vi "LCD string VI.vi"(0 "Error In":errorcluster, 1 "Tank Level (L)":dbl, 3 "1 - cm\n2 - L":dbl=1.0 min=1.0 max=2.0) -> ()   [LabVIEW 2017]
uses:
  <vilib>/MakerHub/LINX/Public/Utilities/Open Serial.vi
  <vilib>/MakerHub/LINX/LMH-LINX.lvlib
panel:
  out "Centimeters":dbl
  in  "stop":bool
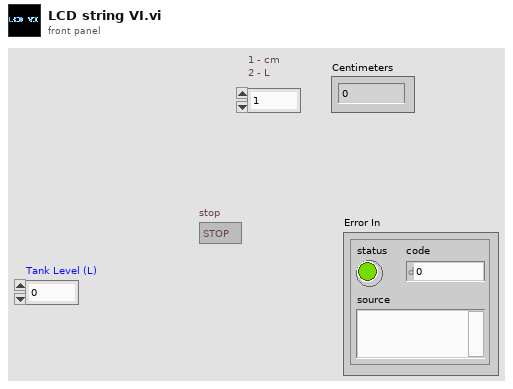
[diagram p1: front panel]
types:
  T1 = typedef "LMH-LINX.lvlib/LINX Ref.ctl" = cluster{"IO":T2, "Interface":T3, "LINX Device Config":T4}
  T2 = typedef "LMH-LINX.lvlib/Platform.ctl" = enum16{"Remote", "Local"}
  T3 = typedef "LMH-LINX.lvlib/Interface.ctl" = enum16{"Serial", "TCP"}
  T4 = typedef "LMH-LINX.lvlib/Device.lvlib/LINX Device Config.ctl" = cluster{"Interface":T3, "COM Port":refnum<visa-resource-name>, "TCP Configuration":T5, "Device Family":u8, "Device ID":u8, "Device Name":string, "TCP Ref":refnum<k5>, "Channels":T6}
  T5 = typedef "LMH-LINX.lvlib/Device.lvlib/TCP Config.ctl" = cluster{"IP Address":string, "Port":u16}
  T6 = typedef "LMH-LINX.lvlib/Channels.ctl" = cluster{"DI":u8[], "DO":u8[], "AI":u8[], "AO":u8[], "PWM":u8[], "QE":u8[], "UART":u8[], "I2C 2":u8[], "SPI":u8[], "CAN":u8[], "Servo":u8[], "AI Ref (V)":dbl, "AI Resolution (Bits)":u8, "AO Ref (V)":dbl, "AO Resolution (Bits)":u8}
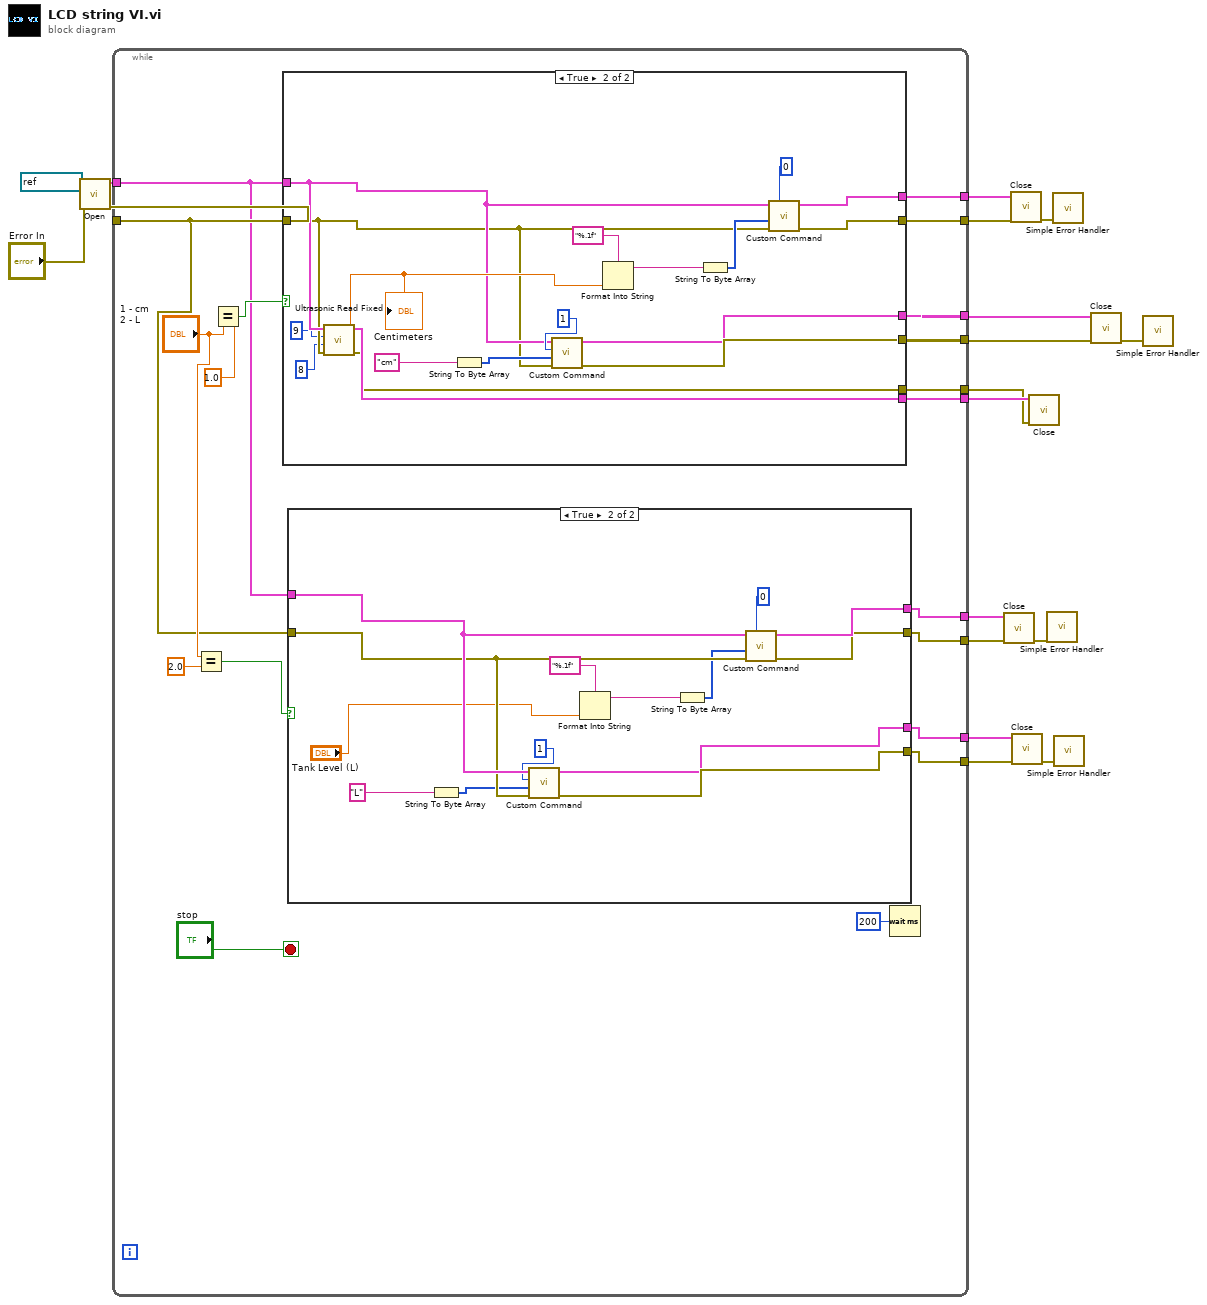
[diagram p0: block diagram]
diagram:
  n1 = call-poly <vilib>:"Open.vi"("Error In"="Error In", "Serial Port"=refnum<visa-resource-name> "COM7") -> ("Error Out"=w15:errorcluster, "LINX Resource"=w14:T1)  [unwired: 7 in, 1 out]
  n2 = while {
    tunnel: w14 -> [w26]
    tunnel: w15 -> [w25]
    tunnel: [w37] -> w18
    tunnel: [w36] -> w17
    tunnel: [w35] -> w12
    tunnel: [w34] -> w11
    tunnel: [w24] -> w8
    tunnel: [w23] -> w7
    tunnel: [w22] -> w6
    tunnel: [w21] -> w5
    tunnel: [w20] -> w2
    tunnel: [w19] -> w1
    stop <- "stop" stop-if-true
    n3 = Equal?(x="1 - cm\n2 - L", y=2.0) -> (x = y?=w27:bool)
    n4 = Equal?(x="1 - cm\n2 - L", y=1.0) -> (x = y?=w30:bool)
    n5 = case shown="True" w30 {
      tunnel: w26 -> [w55 w61]
      tunnel: w25 -> [w54 w60]
      tunnel: [w55 w73] -> w37
      tunnel: [w54 w72] -> w36
      tunnel: [w54 w71] -> w35
      tunnel: [w55 w70] -> w34
      tunnel: [w55 w59] -> w20
      tunnel: [w54 w58] -> w19
      frame False {
      }
      frame True {
        n6 = call "Ultrasonic Read Fixed.vi"("Error In"=w60, "DO Channel"=u8 8, "DI Channel"=u8 9, "LINX Resource"=w61) -> ("Error Out"=w58:errorcluster, "Centimeters"=w62:dbl, "LINX Resource"=w59:T1)  [unwired: 4 in, 1 out]
        "Centimeters" <- w62
        n7 = String To Byte Array(string="cm") -> (unsigned byte array=w66:u8[])
        n8 = call <vilib>:"Custom Command.vi"("Error In"=w60, "Data"=w66, "Custom Command Number"=u16 1, "LINX Resource"=w61) -> ("Error Out"=w71:errorcluster, "LINX Resource"=w70:T1)  [unwired: 4 in, 2 out]
        n9 = Format Into String(format string="%.1f", w62) -> (resulting string=w68:string)  [unwired: 2 in, 1 out]
        n10 = String To Byte Array(string=w68) -> (unsigned byte array=w67:u8[])
        n11 = call <vilib>:"Custom Command.vi"("Error In"=w60, "Data"=w67, "Custom Command Number"=u16 0, "LINX Resource"=w61) -> ("Error Out"=w72:errorcluster, "LINX Resource"=w73:T1)  [unwired: 4 in, 2 out]
      }
    }
    n12 = case shown="True" w27 {
      tunnel: w26 -> [w39 w53]
      tunnel: w25 -> [w38 w52]
      tunnel: [w39 w51] -> w24
      tunnel: [w38 w50] -> w23
      tunnel: [w38 w49] -> w21
      tunnel: [w39 w48] -> w22
      frame False {
      }
      frame True {
        n13 = String To Byte Array(string="L") -> (unsigned byte array=w44:u8[])
        n14 = call <vilib>:"Custom Command.vi"("Error In"=w52, "Data"=w44, "Custom Command Number"=u16 1, "LINX Resource"=w53) -> ("Error Out"=w49:errorcluster, "LINX Resource"=w48:T1)  [unwired: 4 in, 2 out]
        n15 = Format Into String(format string="%.1f", "Tank Level (L)") -> (resulting string=w46:string)  [unwired: 2 in, 1 out]
        n16 = String To Byte Array(string=w46) -> (unsigned byte array=w45:u8[])
        n17 = call <vilib>:"Custom Command.vi"("Error In"=w52, "Data"=w45, "Custom Command Number"=u16 0, "LINX Resource"=w53) -> ("Error Out"=w50:errorcluster, "LINX Resource"=w51:T1)  [unwired: 4 in, 2 out]
      }
    }
    n18 = Wait (ms)(milliseconds to wait=u32 200) -> ()  [unwired: 1 out]
  }
  n19 = call <vilib>:"Close.vi"("Error In"=w7, "LINX Resource"=w8) -> ("Error Out"=w10:errorcluster)  [unwired: 9 in]
  n20 = call <vilib>:"Close.vi"("Error In"=w17, "LINX Resource"=w18) -> ("Error Out"=w16:errorcluster)  [unwired: 9 in]
  n21 = call <vilib>:"Close.vi"("Error In"=w5, "LINX Resource"=w6) -> ("Error Out"=w9:errorcluster)  [unwired: 9 in]
  n22 = call <vilib>:"Close.vi"("Error In"=w1, "LINX Resource"=w2) -> ()  [unwired: 9 in, 1 out]
  n23 = call <vilib>:"Simple Error Handler.vi"("error in (no error)"=w10) -> ()  [unwired: 4 in, 5 out]
  n24 = call <vilib>:"Simple Error Handler.vi"("error in (no error)"=w16) -> ()  [unwired: 4 in, 5 out]
  n25 = call <vilib>:"Simple Error Handler.vi"("error in (no error)"=w9) -> ()  [unwired: 4 in, 5 out]
  n26 = call <vilib>:"Close.vi"("Error In"=w12, "LINX Resource"=w11) -> ("Error Out"=w13:errorcluster)  [unwired: 9 in]
  n27 = call <vilib>:"Simple Error Handler.vi"("error in (no error)"=w13) -> ()  [unwired: 4 in, 5 out]
